vi "Initialize.vi"(5 "Device":string, 7 "INI File Path":path, 9 "PPLs Folder Path":path, 11 "error in":errorcluster) -> (4 "Laser out":refnum<class "Laser.lvclass">, 15 "error out":errorcluster)   [LabVIEW 2018, in "Laser.lvlib" / "Laser.lvclass"]
uses:
  Laser.lvclass
  Laser.lvclass/Laser.ctl
  PPLs/Configuration/Configuration.lvlibp/Configuration.lvclass
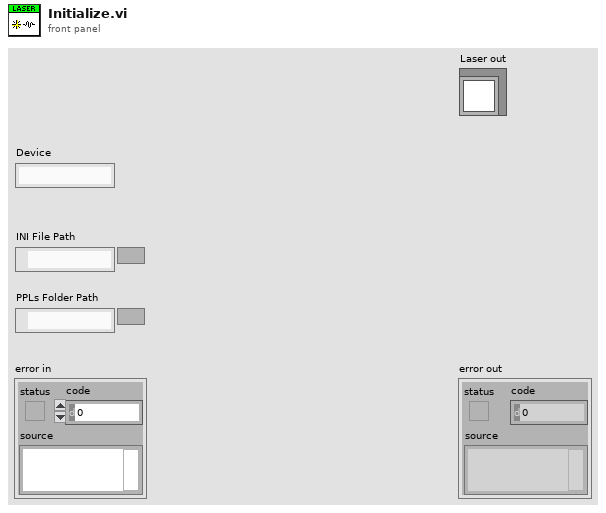
[diagram p1: front panel]
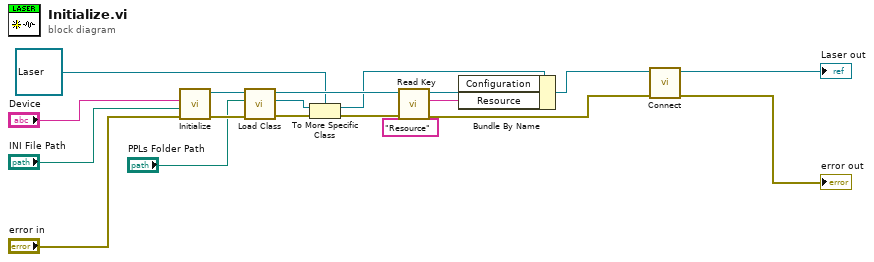
[diagram p0: block diagram]
diagram:
  n1 = call "Initialize.vi"("error in"="error in", "INI File Path"="INI File Path", "Device"="Device") -> ("error out"=w9:errorcluster, "Configuration out"=w19:refnum<class "Configuration.lvclass">)  [unwired: 7 in]
  n2 = call "Load Class.vi"("error in"=w9, "PPLs Folder Path"="PPLs Folder Path", "Configuration in"=w19) -> ("error out"=w16:errorcluster, "Class out"=w17:refnum<class>, "Configuration out"=w18:refnum<class "Configuration.lvclass">)  [unwired: 6 in]
  n3 = To More Specific Class(target class=refnum<class "Laser.lvclass"> refnum ("Laser in"), reference=w17, error in=w16) -> (specific class reference=w13:refnum<class "Laser.lvclass">, error out=w15:errorcluster)
  n4 = call "Read Key.vi"("Key:"="Resource", "error in"=w15, "Configuration in"=w18) -> ("error out"=w6:errorcluster, "Value"=w11:string, "Configuration out"=w12:refnum<class "Configuration.lvclass">)  [unwired: 6 in]
  n5 = Bundle By Name(cluster=w13, "Configuration"=w12, "Resource"=w11) -> (w10:refnum<class "Laser.lvclass">)
  n6 = call-dynamic "Connect.vi"("error in (no error)"=w6, "Laser in"=w10) -> ("error out"=→"error out":errorcluster, "Laser out"=→"Laser out":refnum<class "Laser.lvclass">)  [unwired: 8 in]
